vi "Bin Data.vi"(8 "error in (no error)":errorcluster, 10 "Data in":dbl[][](array[numeric]), 11 "Bin Average in":refnum<class "Bin Average.lvclass">) -> (0 "error out":errorcluster, 3 "Bin Average out":refnum<class "Bin Average.lvclass">)   [LabVIEW 2016, in "Bin Average.lvclass"]
uses:
  Bin Average.lvclass
  Bin Average.lvclass/Bin Average.ctl
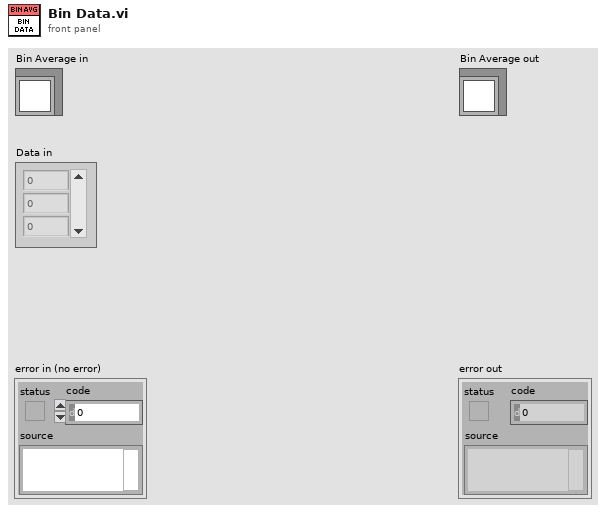
[diagram p1: front panel]
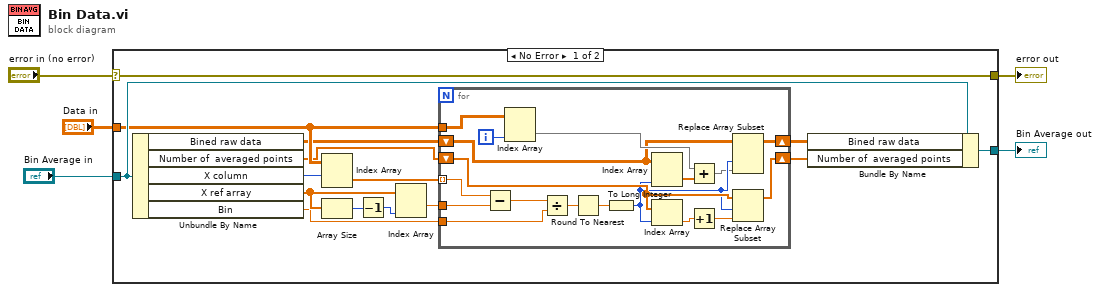
[diagram p0: block diagram]
diagram:
  n1 = case shown="No Error" "error in (no error)" {
    selector: "error in (no error)" -> [w20 w40]
    tunnel: [w20 w40] -> w4
    tunnel: [w9 w39] -> w2
    tunnel: "Bin Average in" -> [w19 w39]
    tunnel: "Data in" -> [w11 _]
    frame No Error {
      n2 = Unbundle By Name(w19) -> ("Bined raw data"=w10:dbl[][], "Number of  averaged points"=w6:dbl[], "X column"=w18:i32, "X ref array"=w16:dbl[], "Bin"=w12:dbl)
      n3 = Index Array(array=w11, index (row)=w18) -> (element=w17:dbl[])  [unwired: 1 in]
      n4 = Array Size(array=w16) -> (size(s)=w15:i32)
      n5 = Decrement(x=w15) -> (x-1=w14:i32)
      n6 = Index Array(array=w16, index #2=w14) -> (element #1=w13:dbl)  [unwired: 1 in, 1 out]
      n7 = for {
        tunnel: w17 -> [w23] mode=indexing
        shift-right: [w31] -> w8
        shift-left: w10 -> [w32]
        tunnel: w11 -> [w38]
        tunnel: w12 -> [w36]
        tunnel: w13 -> [w22]
        shift-right: [w30] -> w7
        shift-left: w6 -> [w29]
        i -> [w37]
        n8 = Subtract(x=w23, y=w22) -> (x-y=w24:dbl)
        n9 = Index Array(array=w38, index (col)=w37) -> (element=w34:dbl[])  [unwired: 1 in]
        n10 = Divide(x=w24, y=w36) -> (x/y=w35:dbl)
        n11 = Round To Nearest(number=w35) -> (nearest integer value=w21:dbl)
        n12 = To Long Integer(number=w21) -> (32bit integer=w27:i32)
        n13 = Index Array(array=w32, index (col)=w27) -> (element=w26:dbl[])  [unwired: 1 in]
        n14 = Index Array(array=w29, index=w27) -> (element=w33:dbl)
        n15 = Add(x=w34, y=w26) -> (x+y=w25:dbl[])
        n16 = Increment(x=w33) -> (x+1=w28:dbl)
        n17 = Replace Array Subset(array=w32, new element=w25, index (col)=w27) -> (w31:dbl[][])  [unwired: 1 in]
        n18 = Replace Array Subset(array=w29, new element=w28, index=w27) -> (w30:dbl[])
      }
      n19 = Bundle By Name(cluster=w19, "Bined raw data"=w8, "Number of  averaged points"=w7) -> (w9:refnum<class "Bin Average.lvclass">)
    }
    frame Error {
    }
  }
  "error out" <- w4
  "Bin Average out" <- w2
